vi "TransformGuassianBlob.vi"(10 "Stretching":T1=[[2.0, 0.0], [0.0, 1.0]], 11 "Rotate":dbl) -> (3 "Blob":dbl[][](array[numeric]))   [LabVIEW 2017]
uses:
  <vilib>/Analysis/Matrix/Datatypes/RealMatrix.ctl
  <vilib>/Analysis/baseanly.llb/Real A x B.vi
  <vilib>/Analysis/baseanly.llb/A x Vector.vi
  <vilib>/Analysis/NI_AALBase.lvlib
  <vilib>/Analysis/Matrix/NI_Matrix.lvlib
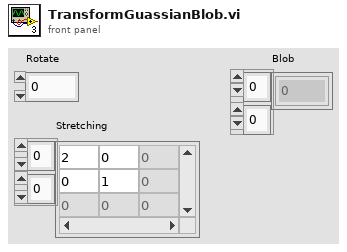
[diagram p1: front panel]
types:
  T1 = typedef "NI_Matrix.lvlib/RealMatrix.ctl" = dbl[][]
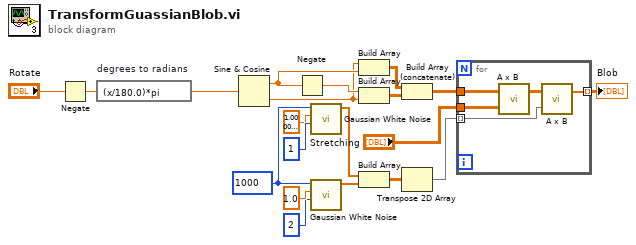
[diagram p0: block diagram]
diagram:
  w5 = 1000 ("samples")
  n1 = Negate(x="Rotate") -> (-x=w19:dbl)
  n2 = expression code="(x/180.0)*pi" "degrees to radians"(w19) -> (w11:dbl)
  n3 = Sine & Cosine(0:w11) -> (1:w16:dbl, 2:w14:dbl)
  n4 = Negate(x=w16) -> (-x=w15:dbl)
  n5 = call <vilib>:"Gaussian White Noise.vi"("seed"=1, "standard deviation"=1.0000000000000002, "samples"=w5) -> ("Gaussian noise pattern"=w9:dbl[])  [unwired: 7 in, 1 out]
  n6 = call <vilib>:"Gaussian White Noise.vi"("seed"=2, "standard deviation"=1.0, "samples"=w5) -> ("Gaussian noise pattern"=w10:dbl[])  [unwired: 7 in, 1 out]
  n7 = Build Array(w14, w16) -> (w12:T1)
  n8 = Build Array(w15, w14) -> (w13:T1)
  n9 = Build Array(w9, w10) -> (w6:dbl[][])
  n10 = Build Array (concatenate)(w12, w13) -> (w17:T1)
  n11 = Transpose 2D Array(2D array=w6) -> (transposed array=w20:dbl[][])
  n12 = for {
    tunnel: w20 -> [w25] mode=indexing
    tunnel: "Stretching" -> [w23]
    tunnel: [w24] -> w8 mode=indexing
    tunnel: w17 -> [w22]
    n13 = call-poly <vilib>:"A x B.vi"("B"=w23, "A"=w22) -> ("A x B"=w21:T1)  [unwired: 1 out]
    n14 = call-poly <vilib>:"A x B.vi"("Vector"=w25, "A"=w21) -> ("A x Vector"=w24:dbl[])  [unwired: 1 out]
  }
  "Blob" <- w8
